vi "Get VI Name.vi"(8 "error in (no error)":errorcluster) -> (0 "error out":errorcluster, 3 "VI Name":string)   [LabVIEW 2014, in "SLL Application.lvlib"]
doc: "Get the unique name of the VI. \n\nThis would return the VI name if the VI is non-reentrant and would return the clone name when the VI is re-entrant."
uses:
  SLL Application.lvlib
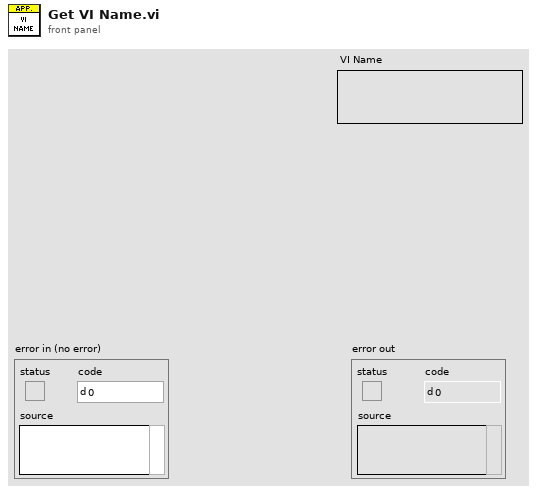
[diagram p1: front panel]
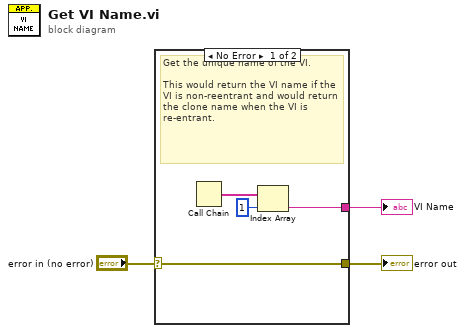
[diagram p0: block diagram]
diagram:
  n1 = case shown="No Error" "error in (no error)" {
    selector: "error in (no error)" -> [w7 w8]
    tunnel: [w7 w8] -> w2
    tunnel: [w4 _] -> w1
    frame No Error {
      # "Get the unique name of the VI. \n\nThis would return the VI name if the VI is non-reentrant and would return the clone name when the VI is re-entrant."
      n2 = Call Chain() -> (call chain=w6:string[])
      n3 = Index Array(array=w6, index=1) -> (element=w4:string)
    }
    frame Error {
    }
  }
  "error out" <- w2
  "VI Name" <- w1
